vi "Read NTCs.vi"(6 "error in":errorcluster, 8 "MaxRead":i32, 9 "Channel in":u16) -> (0 "error out":errorcluster, 1 "Messages":T1(array[cluster]), 2 "Pass":bool, 3 "Channel out":u16)   [LabVIEW 2023]
uses:
  4f930f32-d09a-43ef-bca1-8b214b378bd5.vi
  e8470de1-fa2d-4ee3-b50e-96bd89dc731f.vi
  d0f02419-cfb7-4a5e-bc3c-f035efdb0e96.vi
  Communication/PCAN2023/PCAN API.lvlib
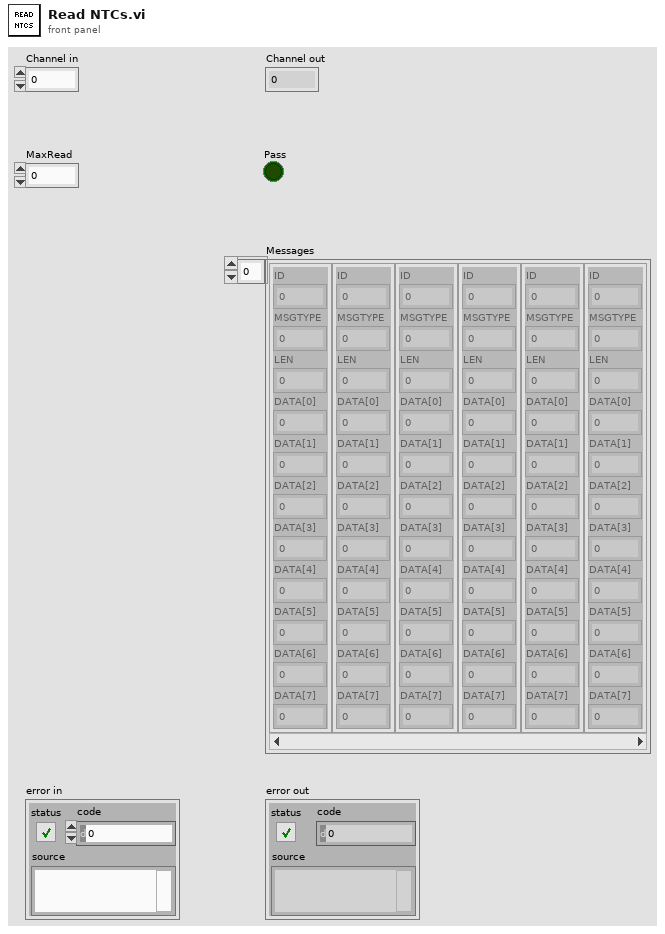
[diagram p1: front panel]
types:
  T1 = cluster{"ID":u32, "MSGTYPE":u8, "LEN":u8, "DATA[0]":u8, "DATA[1]":u8, "DATA[2]":u8, "DATA[3]":u8, "DATA[4]":u8, "DATA[5]":u8, "DATA[6]":u8, "DATA[7]":u8}[]
  T2 = cluster{"ID":u32, "MSGTYPE":u8, "LEN":u8, "DATA[0]":u8, "DATA[1]":u8, "DATA[2]":u8, "DATA[3]":u8, "DATA[4]":u8, "DATA[5]":u8, "DATA[6]":u8, "DATA[7]":u8}
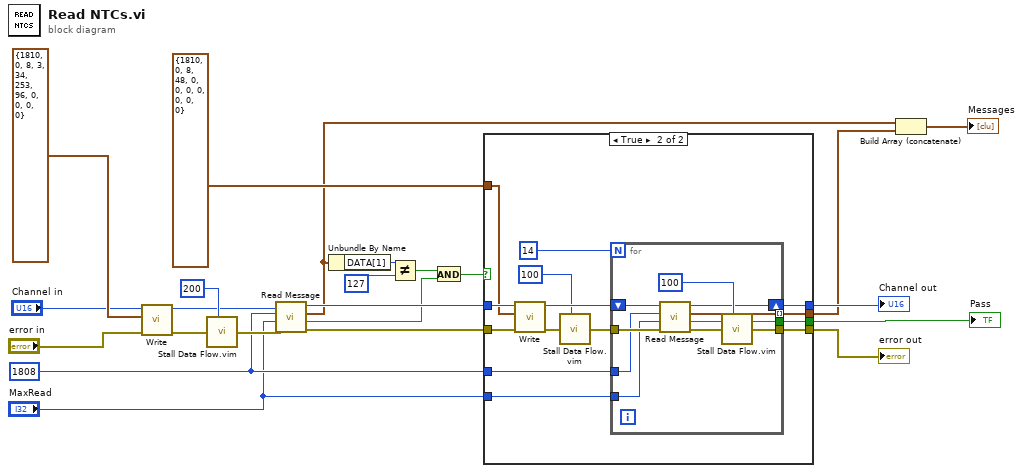
[diagram p0: block diagram]
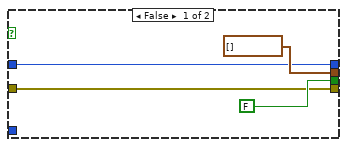
[diagram p2: hidden frame]
diagram:
  (unwired) u32 200 ("milliseconds to wait")
  w2 = u32 1808 ("ID")
  n1 = call "Write.vi"("error in"="error in", "MessageBuffer"=T2 {"ID"=1810, "MSGTYPE"=0, "LEN"=8, "DATA[0]"=3, "DATA[1]"=34, "DATA[2]"=253, "DATA[3]"=96, "DATA[4]"=0, "DATA[5]"=0, "DATA[6]"=0, "DATA[7]"=0}, "Channel"="Channel in") -> ("error out"=w19:errorcluster, "Channel out"=w11:u16)  [unwired: 5 in, 2 out]
  n2 = call "Stall Data Flow.vim"("value in"=w19, "milliseconds to wait"=u32 200) -> ("value out"=w7:errorcluster)  [unwired: 1 out]
  n3 = call "Read Message.vi"("error in"=w7, "MaxRead"="MaxRead", "ID"=w2, "Channel in"=w11) -> ("error out"=w8:errorcluster, "Passed"=w5:bool, "Last Message"=w9:T2, "Channel out"=w10:u16)  [unwired: 3 in, 1 out]
  n4 = Unbundle By Name(w9) -> ("DATA[1]"=w15:u8)
  n5 = Not Equal?(x=w15, y=u8 127) -> (x != y?=w6:bool)
  n6 = And(x=w6, y=w5) -> (x .and. y?=w4:bool)
  n7 = case shown="True" w4 {
    tunnel: w10 -> [w26 w41]
    tunnel: w8 -> [w24 w40]
    tunnel: [w24 w39] -> w18
    tunnel: [FALSE w38] -> w3
    tunnel: [w26 w36] -> w17
    tunnel: T2 {"ID"=1810, "MSGTYPE"=0, "LEN"=8, "DATA[0]"=48, "DATA[1]"=0, "DATA[2]"=0, "DATA[3]"=0, "DATA[4]"=0, "DATA[5]"=0, "DATA[6]"=0, "DATA[7]"=0} ("MessageBuffer") -> [_ w34]
    tunnel: [T1 [] w30] -> w13
    tunnel: w2 -> [_ w29]
    tunnel: "MaxRead" -> [_ w28]
    frame False {
    }
    frame True {
      n8 = call "Write.vi"("error in"=w40, "MessageBuffer"=w34, "Channel"=w41) -> ("error out"=w31:errorcluster, "Channel out"=w37:u16)  [unwired: 5 in, 2 out]
      n9 = call "Stall Data Flow.vim"("value in"=w31, "milliseconds to wait"=u32 100) -> ("value out"=w35:errorcluster)  [unwired: 1 out]
      n10 = for {
        N: 14 -> [_]
        tunnel: [w44] -> w38
        shift-right: [w48] -> w36
        shift-left: w37 -> [w49]
        tunnel: w35 -> [w47]
        tunnel: [w51] -> w39
        tunnel: [w45] -> w30 mode=indexing
        tunnel: w29 -> [w43]
        tunnel: w28 -> [w42]
        n11 = call "Read Message.vi"("error in"=w47, "MaxRead"=w42, "ID"=w43, "Channel in"=w49) -> ("error out"=w46:errorcluster, "Passed"=w44:bool, "Last Message"=w45:T2, "Channel out"=w48:u16)  [unwired: 3 in, 1 out]
        n12 = call "Stall Data Flow.vim"("value in"=w46, "milliseconds to wait"=u32 100) -> ("value out"=w51:errorcluster)  [unwired: 1 out]
      }
    }
  }
  "error out" <- w18
  "Channel out" <- w17
  "Pass" <- w3
  n13 = Build Array (concatenate)(w9, w13) -> (→"Messages":T1)
